vi "Agilent N6700 Series Configure Voltage.vi"() -> ()   [LabVIEW 2021]
doc: "Configures the power supply's output range on a channel, configures the DC voltage level, channel appears at the output connector and takes a measurement on the output signal and returns the measured value."
uses:
  <instrlib>/Agilent 3446X Series/Public/Data/Read (Single Point).vi
  <instrlib>/Agilent N6700 Series/Agilent N6700 Series.lvlib
  <instrlib>/Agilent 3446X Series/Agilent 3446X Series.lvlib
panel:
  out "DMM Current Measurement":dbl
  in  "Current Manual Range (1)":dbl=1.0
  in  "Agilent DMM Current":refnum<visa-resource-name>
  out "DMM Voltage Measurement":dbl
  in  "Voltage Manual Range (1)":dbl=1.0
  in  "Agilent DMM Voltage":refnum<visa-resource-name>
  in  "Absolute Resolution":dbl=1e-06
  in  "error in":errorcluster {"code" format="%.0x"}
  out "error out":errorcluster {"code" format="%.0x"}
  in  "Load Current Limit":dbl=1.0 format="%^.3e"
  in  "Load Behavior":i32(ring) items=["Regulatory Limit", "Trip Limit"]
  out "Load Voltage Measurement":dbl format="%^.3e"
  in  "Load Voltage Level":dbl=5.0 format="%^.3e"
  in  "Load Voltage Range":dbl=10.0 format="%^.3e"
  in  "Load SMUChannel":string="1"
  in  "Load SMU":refnum<visa-resource-name>
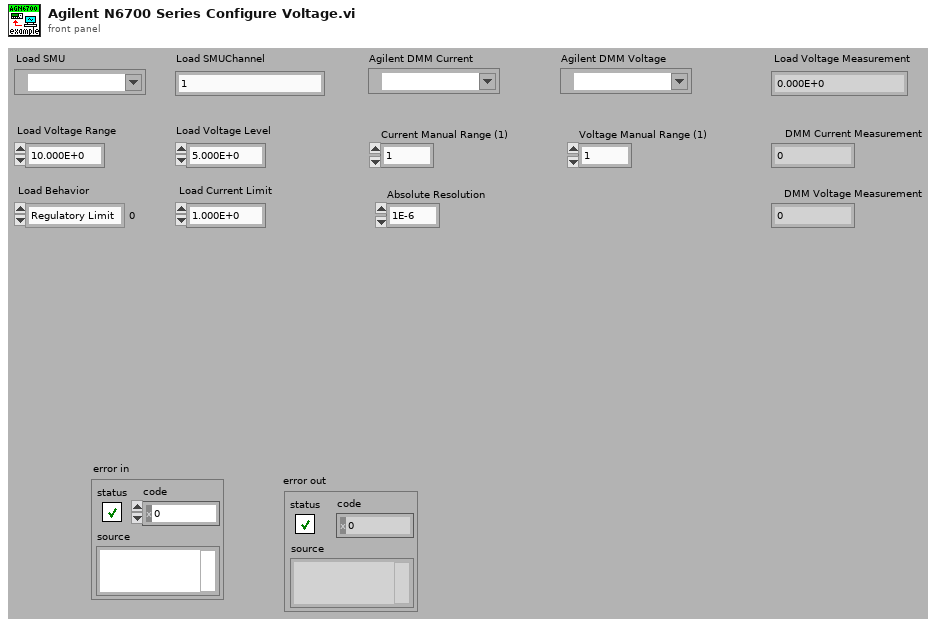
[diagram p1: front panel]
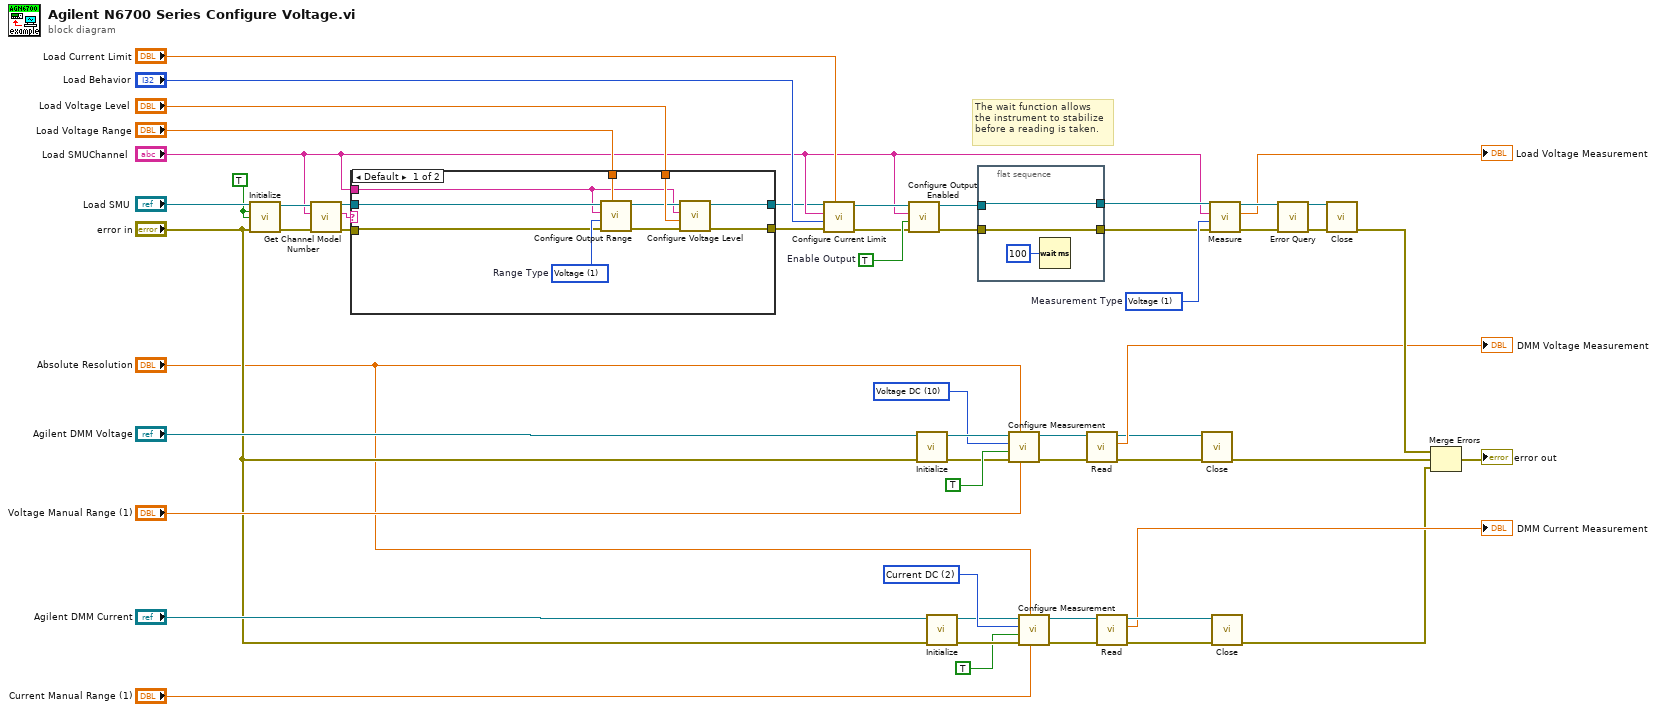
[diagram p0: block diagram]
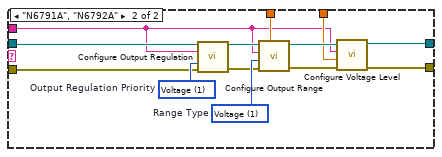
[diagram p2: hidden frame]
diagram:
  w14 = 2 items=["Continuity", "Current AC", "Current DC", "Diode", "Frequency", "Resistance 4-wire", "Period", "Resistance 2-wire", "Temperature", "Voltage AC", "Voltage DC", "Voltage DC Ratio", "Capacitance"] ("Measurement Function (10: Voltage DC)")
  w15 = 10 items=["Continuity", "Current AC", "Current DC", "Diode", "Frequency", "Resistance 4-wire", "Period", "Resistance 2-wire", "Temperature", "Voltage AC", "Voltage DC", "Voltage DC Ratio", "Capacitance"] ("Measurement Function (10: Voltage DC)")
  w46 = TRUE ("Reset? (T: Yes)")
  w47 = 1 items=["Voltage"=1, "Current"=0]  # Measurement Type
  w48 = TRUE  # Enable Output
  # "The wait function allows \nthe instrument to stabilize\nbefore a reading is taken."
  n1 = call <instrlib>:"Initialize.vi"("VISA resource name"="Load SMU", "ID Query? (T: Yes)"=w46, "Reset? (T: Yes)"=w46, "error in (no error)"="error in") -> ("VISA resource name out"=w37:refnum<visa-resource-name>, "error out"=w36:errorcluster)  [unwired: 10 in]
  n2 = call <instrlib>:"Get Channel Model Number.vi"("error in (no error)"=w36, "Channel Name (1)"="Load SMUChannel", "VISA resource name"=w37) -> ("error out"=w34:errorcluster, "Model Number"=w33:string, "VISA resource name out"=w35:refnum<visa-resource-name>)  [unwired: 6 in]
  n3 = case shown="Default" w33 {
    tunnel: "Load Voltage Range" -> [w62 w78]
    tunnel: "Load SMUChannel" -> [w56 w68]
    tunnel: w35 -> [w64 w73]
    tunnel: w34 -> [w63 w72]
    tunnel: "Load Voltage Level" -> [w60 w69]
    tunnel: [w58 w66] -> w30
    tunnel: [w57 w67] -> w29
    frame Default {
      w65 = 1 items=["Voltage"=1, "Current"=0]  # Range Type
      n4 = call <instrlib>:"Configure Output Range.vi"("Range (0.0)"=w62, "error in (no error)"=w63, "Range Type (1: Voltage)"=w65, "Channel Name (1)"=w56, "VISA resource name"=w64) -> ("error out"=w61:errorcluster, "VISA resource name out"=w59:refnum<visa-resource-name>)  [unwired: 5 in]
      n5 = call <instrlib>:"Configure Voltage Level.vi"("error in (no error)"=w61, "Level  (0.0 volts)"=w60, "Channel Name (1)"=w56, "VISA resource name"=w59) -> ("error out"=w58:errorcluster, "VISA resource name out"=w57:refnum<visa-resource-name>)  [unwired: 6 in]
    }
    frame "N6791A", "N6792A" {
      w74 = 1 items=["Voltage"=1, "Current"=0]  # Output Regulation Priority
      w77 = 1 items=["Voltage"=1, "Current"=0]  # Range Type
      n6 = call <instrlib>:"Configure Output Regulation.vi"("VISA resource name"=w73, "Channel Name (1)"=w68, "Output Regulation Priority (1: Voltage)"=w74, "error in (no error)"=w72) -> ("VISA resource name out"=w76:refnum<visa-resource-name>, "error out"=w75:errorcluster)  [unwired: 10 in]
      n7 = call <instrlib>:"Configure Output Range.vi"("Range (0.0)"=w78, "error in (no error)"=w75, "Range Type (1: Voltage)"=w77, "Channel Name (1)"=w68, "VISA resource name"=w76) -> ("error out"=w70:errorcluster, "VISA resource name out"=w71:refnum<visa-resource-name>)  [unwired: 5 in]
      n8 = call <instrlib>:"Configure Voltage Level.vi"("error in (no error)"=w70, "Level  (0.0 volts)"=w69, "Channel Name (1)"=w68, "VISA resource name"=w71) -> ("error out"=w66:errorcluster, "VISA resource name out"=w67:refnum<visa-resource-name>)  [unwired: 6 in]
    }
  }
  n9 = call <instrlib>:"Configure Current Limit.vi"("Limit (0.0 amps)"="Load Current Limit", "error in (no error)"=w30, "Behavior (0: Regulatory Limit)"="Load Behavior", "Channel Name (1)"="Load SMUChannel", "VISA resource name"=w29) -> ("error out"=w45:errorcluster, "VISA resource name out"=w44:refnum<visa-resource-name>)  [unwired: 5 in]
  n10 = call <instrlib>:"Configure Output Enabled.vi"("error in (no error)"=w45, "Enable Output (False)"=w48, "Channel Name (1)"="Load SMUChannel", "VISA resource name"=w44) -> ("error out"=w38:errorcluster, "VISA resource name out"=w41:refnum<visa-resource-name>)  [unwired: 6 in]
  n11 = call <instrlib>:"Initialize.vi"("error in (no error)"="error in", "VISA resource name"="Agilent DMM Voltage") -> ("error out"=w20:errorcluster, "VISA resource name out"=w19:refnum<visa-resource-name>)  [unwired: 3 in, 5 out]
  n12 = call <instrlib>:"Initialize.vi"("error in (no error)"="error in", "VISA resource name"="Agilent DMM Current") -> ("error out"=w10:errorcluster, "VISA resource name out"=w11:refnum<visa-resource-name>)  [unwired: 3 in, 5 out]
  n13 = flat-sequence {
    tunnel: w41 -> [w81]
    tunnel: [w81] -> w40
    tunnel: [w79] -> w39
    tunnel: w38 -> [w79]
    frame #0 {
      n14 = Wait (ms)(milliseconds to wait=u32 100) -> ()  [unwired: 1 out]
    }
  }
  n15 = call <instrlib>:"Configure Measurement.vi"("Manual Range (1)"="Voltage Manual Range (1)", "Absolute Resolution (1E-6)"="Absolute Resolution", "error in (no error)"=w20, "Auto Range (T: Enable)"=TRUE, "Measurement Function (10: Voltage DC)"=w15, "VISA resource name"=w19) -> ("error out"=w22:errorcluster, "VISA resource name out"=w21:refnum<visa-resource-name>)  [unwired: 4 out]
  n16 = call <instrlib>:"Configure Measurement.vi"("Manual Range (1)"="Current Manual Range (1)", "Absolute Resolution (1E-6)"="Absolute Resolution", "error in (no error)"=w10, "Auto Range (T: Enable)"=TRUE, "Measurement Function (10: Voltage DC)"=w14, "VISA resource name"=w11) -> ("error out"=w8:errorcluster, "VISA resource name out"=w9:refnum<visa-resource-name>)  [unwired: 4 out]
  n17 = call-poly <instrlib>:"Read.vi"("error in (no error)"=w22, "VISA resource name"=w21) -> ("error out"=w17:errorcluster, "Measurement"=→"DMM Voltage Measurement":dbl, "VISA resource name out"=w18:refnum<visa-resource-name>)  [unwired: 7 out]
  n18 = call-poly <instrlib>:"Read.vi"("error in (no error)"=w8, "VISA resource name"=w9) -> ("error out"=w13:errorcluster, "Measurement"=→"DMM Current Measurement":dbl, "VISA resource name out"=w12:refnum<visa-resource-name>)  [unwired: 7 out]
  n19 = call <instrlib>:"Close.vi"("error in (no error)"=w17, "VISA resource name"=w18) -> ("error out"=w16:errorcluster)  [unwired: 9 out]
  n20 = call <instrlib>:"Measure.vi"("error in (no error)"=w39, "Measurement Type (1: Voltage)"=w47, "Channel Name (1)"="Load SMUChannel", "VISA resource name"=w40) -> ("error out"=w55:errorcluster, "Measurement"=→"Load Voltage Measurement":dbl, "VISA resource name out"=w52:refnum<visa-resource-name>)  [unwired: 5 in]
  n21 = call <instrlib>:"Close.vi"("error in (no error)"=w13, "VISA resource name"=w12) -> ("error out"=w3:errorcluster)  [unwired: 9 out]
  n22 = call <instrlib>:"Error Query.vi"("VISA resource name"=w52, "error in (no error)"=w55) -> ("VISA resource name out"=w53:refnum<visa-resource-name>, "error out"=w54:errorcluster)  [unwired: 10 in, 2 out]
  n23 = call <instrlib>:"Close.vi"("VISA resource name"=w53, "error in (no error)"=w54) -> ("error out"=w28:errorcluster)  [unwired: 13 in]
  n24 = Merge Errors(w28, w16, w3) -> (→"error out":errorcluster)
